vi "Turn PID.vi"(10 "Setpoint X":dbl=171.18064895153134, 11 "Current X":dbl=167.0) -> (2 "Aligned?":bool=TRUE, 3 "Motor Out":cluster{"output":dbl, dbl}={"output"=0.20427375144951004, -0.20427375144951004})   [LabVIEW 2011]
uses:
  <vilib>/addons/control/pid/pid.llb/PID (DBL).vi
  <vilib>/addons/control/pid/NI_PID_pid.lvlib
panel:
  in  "dt (s)":dbl=0.02
  in  "output range":cluster{"output high":dbl, "output low":dbl}={"output high"=0.3, "output low"=-0.3}
  out "Waveform Chart":dbl(graph)=4.180648951531339
  in  "PID gains":T1={"proportional gain (Kc)"=0.9, "integral time (Ti, min)"=0.5, "derivative time (Td, min)"=0.0002} {"derivative time (Td, min)" format="%.5f"; "integral time (Ti, min)" format="%.8f"; "proportional gain (Kc)" format="%.5f"}
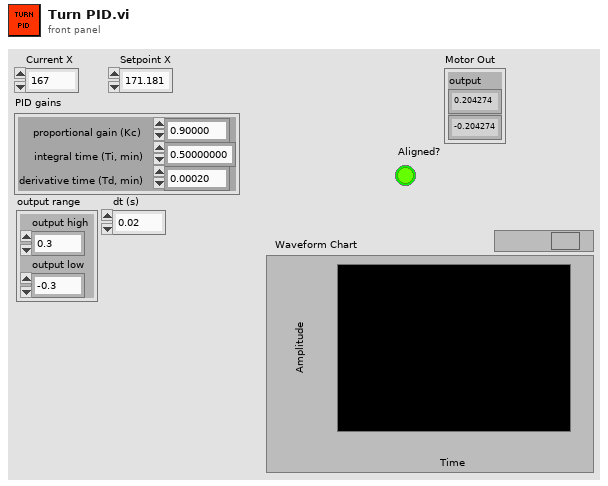
[diagram p1: front panel]
types:
  T1 = cluster{"proportional gain (Kc)":dbl, "integral time (Ti, min)":dbl, "derivative time (Td, min)":dbl}
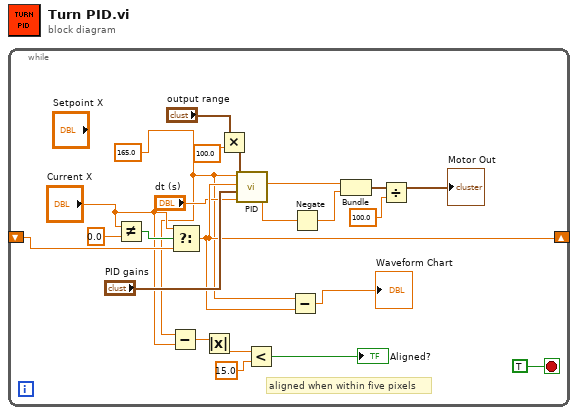
[diagram p0: block diagram]
diagram:
  n1 = while {
    shift-right: [w14] -> _
    shift-left: _ -> [w16]
    stop <- TRUE stop-if-true
    w1 = 165.0
    # "aligned when within five pixels"
    n2 = Not Equal?(x="Current X", y=0.0) -> (x != y?=w17:bool)
    n3 = Subtract(x=w1, y="Current X") -> (x-y=w10:dbl)
    n4 = Select(t="Current X", s=w17, f=w16) -> (s? t:f=w14:dbl)
    n5 = Absolute Value(x=w10) -> (abs(x)=w8:dbl)
    n6 = Multiply(x="output range", y=100.0 ("output low")) -> (x*y=w6:cluster{"output high":dbl, "output low":dbl})
    n7 = call-poly <vilib>:"PID.vi"("output range"=w6, "dt (s)"="dt (s)", "PID gains"="PID gains", "process variable"=w14, "setpoint"=w1) -> ("output"=w13:dbl)  [unwired: 5 in, 1 out]
    n8 = Less?(x=w8, y=15.0) -> (x < y?=→"Aligned?":bool)
    n9 = Subtract(x=w1, y=w14) -> (x-y=→"Waveform Chart":dbl)
    n10 = Negate(x=w13) -> (-x=w20:dbl)
    n11 = Bundle("output"=w13, w20) -> (w12:cluster{"output":dbl, dbl})  [unwired: 1 in]
    n12 = Divide(x=w12, y=100.0 ("output low")) -> (x/y=→"Motor Out":cluster{"output":dbl, dbl})
  }
